vi "多态-列表插入项名.vi"   [LabVIEW 2017]
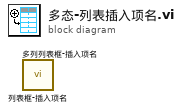
[diagram p0: block diagram]
diagram:
  n1 = call "列表框-插入项名.vi"() -> ()  [unwired: 11 in, 1 out]
  n2 = call "多列列表框-插入项名.vi"() -> ()  [unwired: 11 in, 1 out]
